vi "Write Target Time.vi"(8 "error in (no error)":errorcluster, 10 "Target Time":timestamp, 11 "TimerSensor in":refnum<class "TimerSensorConfig.lvclass">) -> (0 "error out":errorcluster, 3 "TimerSensor out":refnum<class "TimerSensorConfig.lvclass">)   [LabVIEW 2012, in "TimerSensor.lvlib" / "TimerSensorConfig.lvclass"]
uses:
  TimerSensorConfig.lvclass
  TimerSensorConfig.lvclass/TimerSensorConfig.ctl
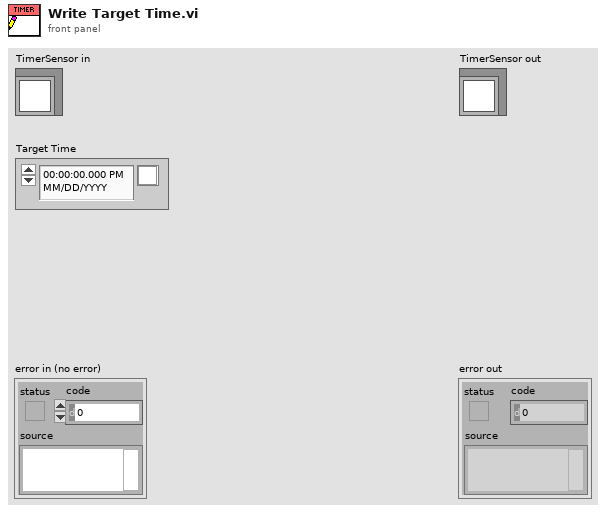
[diagram p1: front panel]
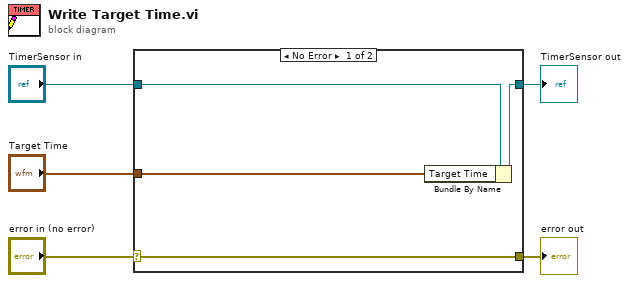
[diagram p0: block diagram]
diagram:
  n1 = case shown="No Error" "error in (no error)" {
    selector: "error in (no error)" -> [w9 w10]
    tunnel: [w9 w10] -> w4
    tunnel: [w7 w11] -> w2
    tunnel: "TimerSensor in" -> [w8 w11]
    tunnel: "Target Time" -> [w6 _]
    frame No Error {
      n2 = Bundle By Name(cluster=w8, "Target Time"=w6) -> (w7:refnum<class "TimerSensorConfig.lvclass">)
    }
    frame Error {
    }
  }
  "error out" <- w4
  "TimerSensor out" <- w2
